vi "TakaData_TMotor_LightField.vi"(0 "Start position Y":dbl, 1 "Start position X":dbl, 2 "TotalSteps Y":i32, 3 "TotalSteps X":i32, 4 "Step Size Y":dbl, 5 "Step Size X":dbl, 7 "min":i32, 9 "max":i32, 10 "TCubeDCServoControl Y":refnum<k24>(container), 12 "TCubeDCServoControl X":refnum<k24>(container), 13 "TOTAL STOP":bool, 19 "Take data":bool) -> (14 "Intensity Graph":dbl[][](graph), 15 "ROI 1, Frame 1, Row 1":dbl[](graph), 16 "Data":T1(array[cluster]))   [LabVIEW 2020]
uses:
  D:/Programs/Fatima/Lightfield-LabVIEW Automation/lightfield-automation-labview/TCube_motion/Kinesis/Thorlabs.MotionControl.Controls.dll
  Kinesis/Thorlabs.MotionControl.Controls.dll
  D:/Programs/Fatima/Lightfield-LabVIEW Automation/lightfield-automation-labview/TCube_motion/Kinesis/Thorlabs.MotionControl.TCube.DCServoCLI.dll
  Kinesis/Thorlabs.MotionControl.TCube.DCServoCLI.dll
  <vilib>/express/express shared/transition.llb/Dynamic To Waveform Array.vi
  <vilib>/express/express signal manip/GetorSetDDTAttributes/Set DDT Attributes/SetT0.vi
  <vilib>/express/express shared/transition.llb/Waveform Array To Dynamic.vi
  <vilib>/express/express signal manip/GetorSetDDTAttributes/Set DDT Attributes/Set DDT Properties.xnode
  LightField Automation.lvclass
panel:
  out "Sums array":dbl[][](array[numeric])
  out "final":dbl[][](array[numeric])
  out "Position Y":i32
  out "Position X":i32
  out "Ys":dbl[](array[numeric])
  out "Xs":dbl[](array[numeric])
  out "sumas":dbl[](array[numeric])
  out "sum":dbl
  in  "SerialNumber X":string="83819717"
  in  "SerialNumber Y":string="83817852"
  # "Range"
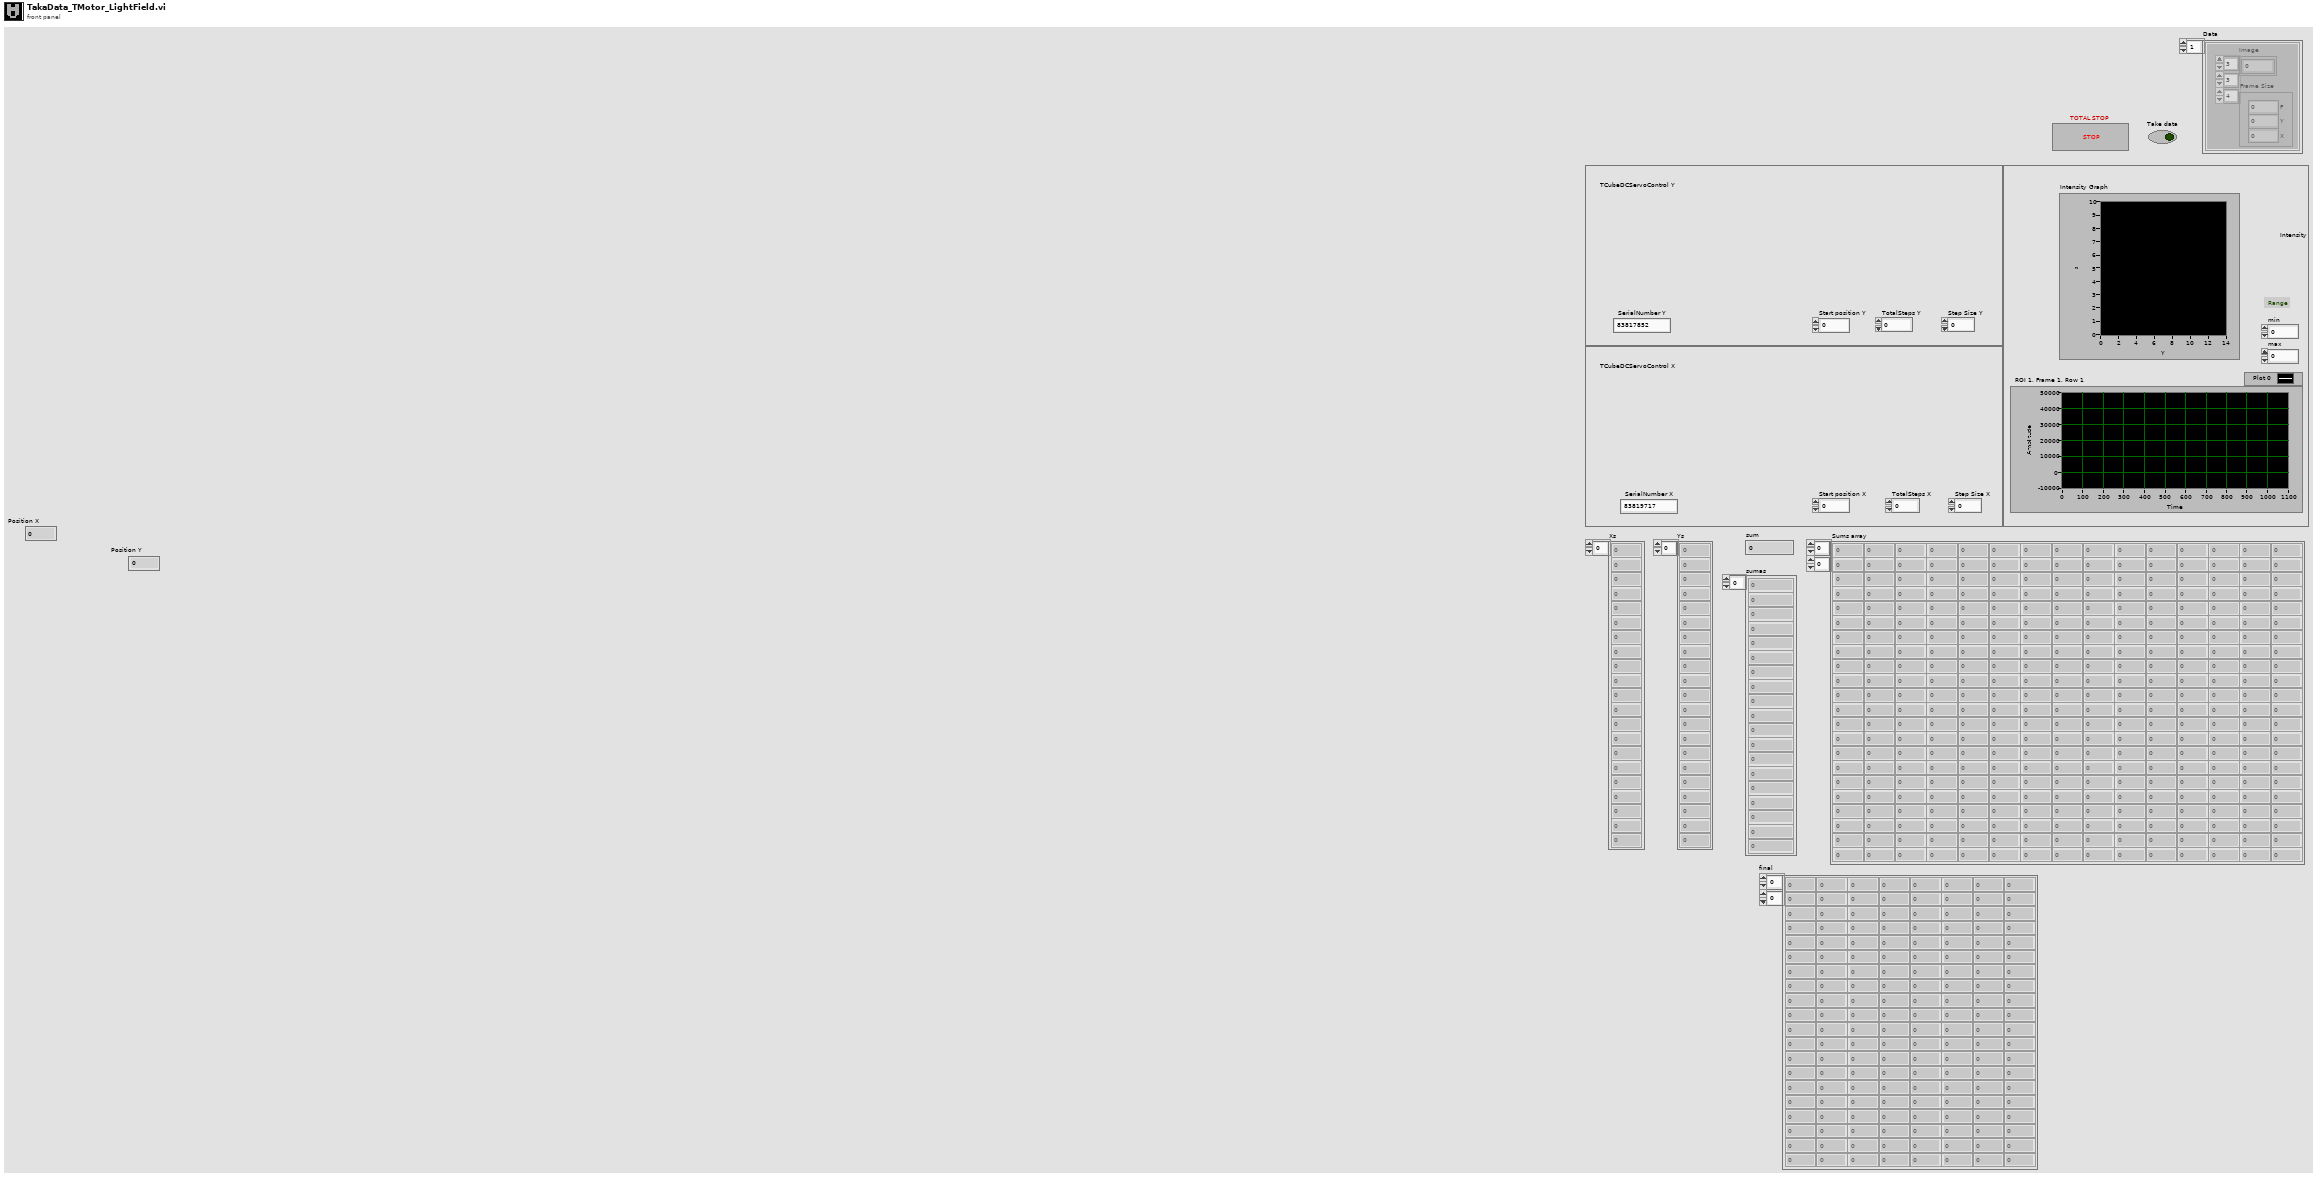
[diagram p1: front panel]
types:
  T1 = cluster{"Image":dbl[][][], "Frame Size":cluster{"F":i32, "Y":i32, "X":i32}}[]
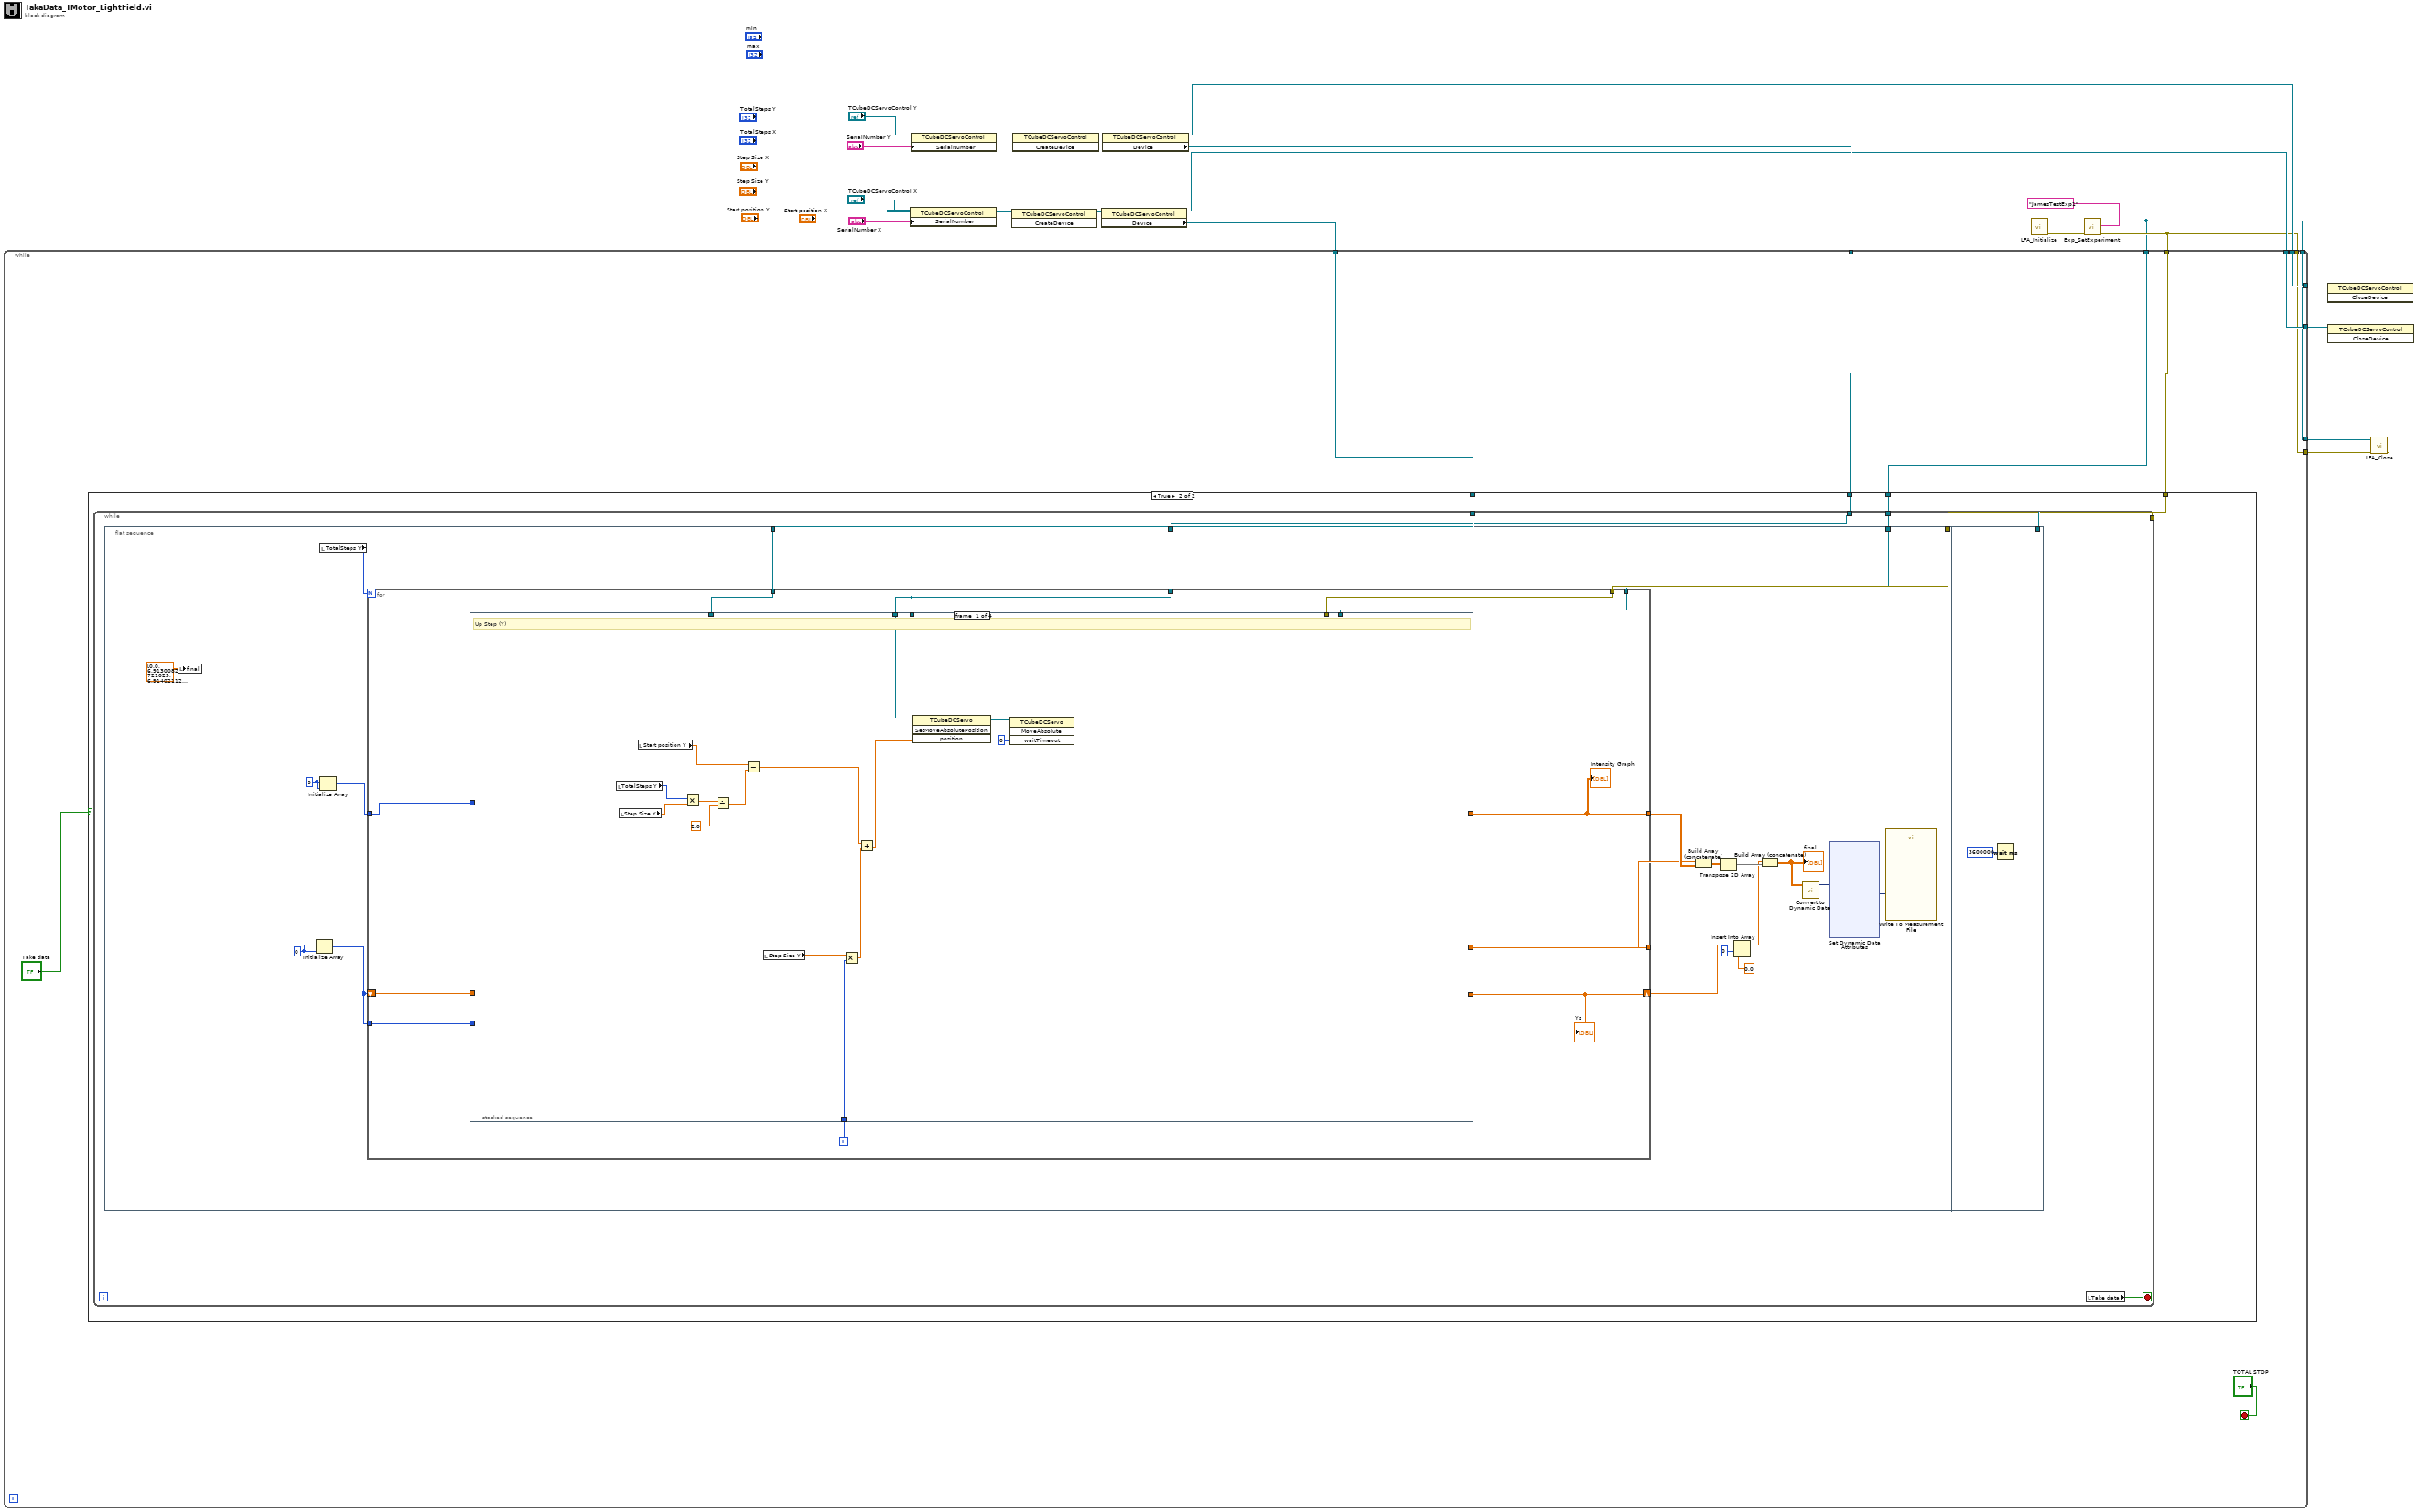
[diagram p0: block diagram]
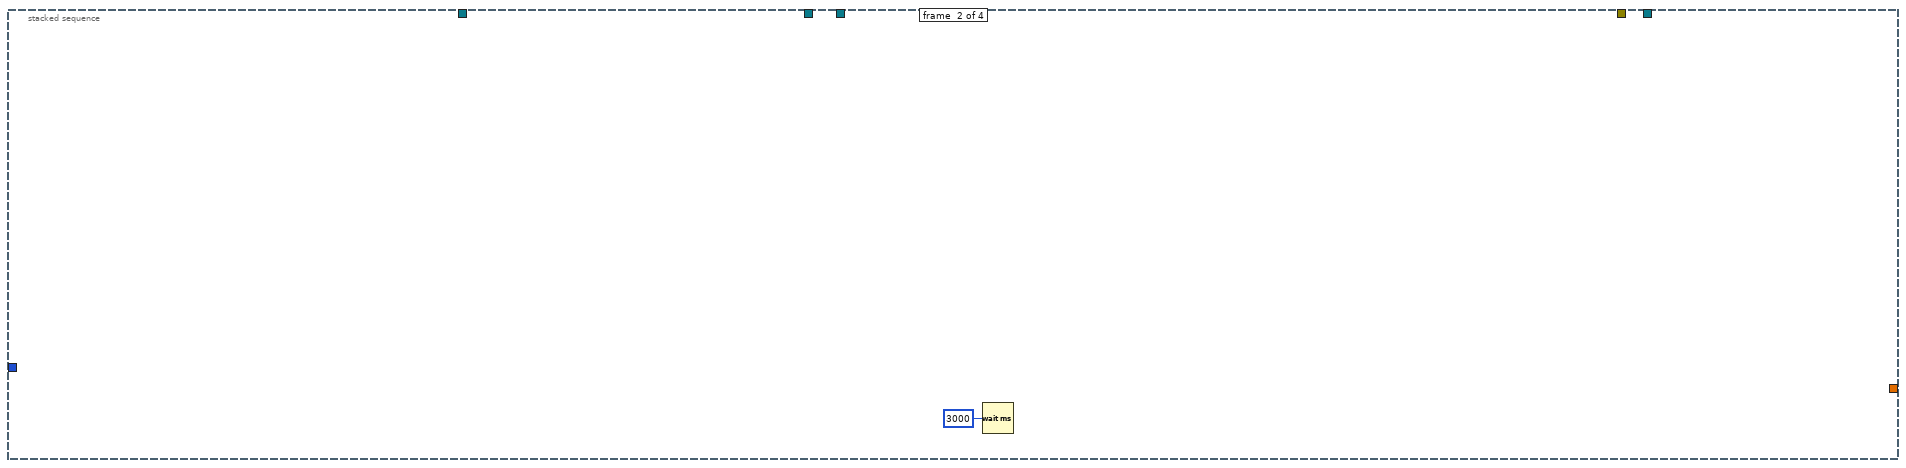
[diagram p3: hidden frame]
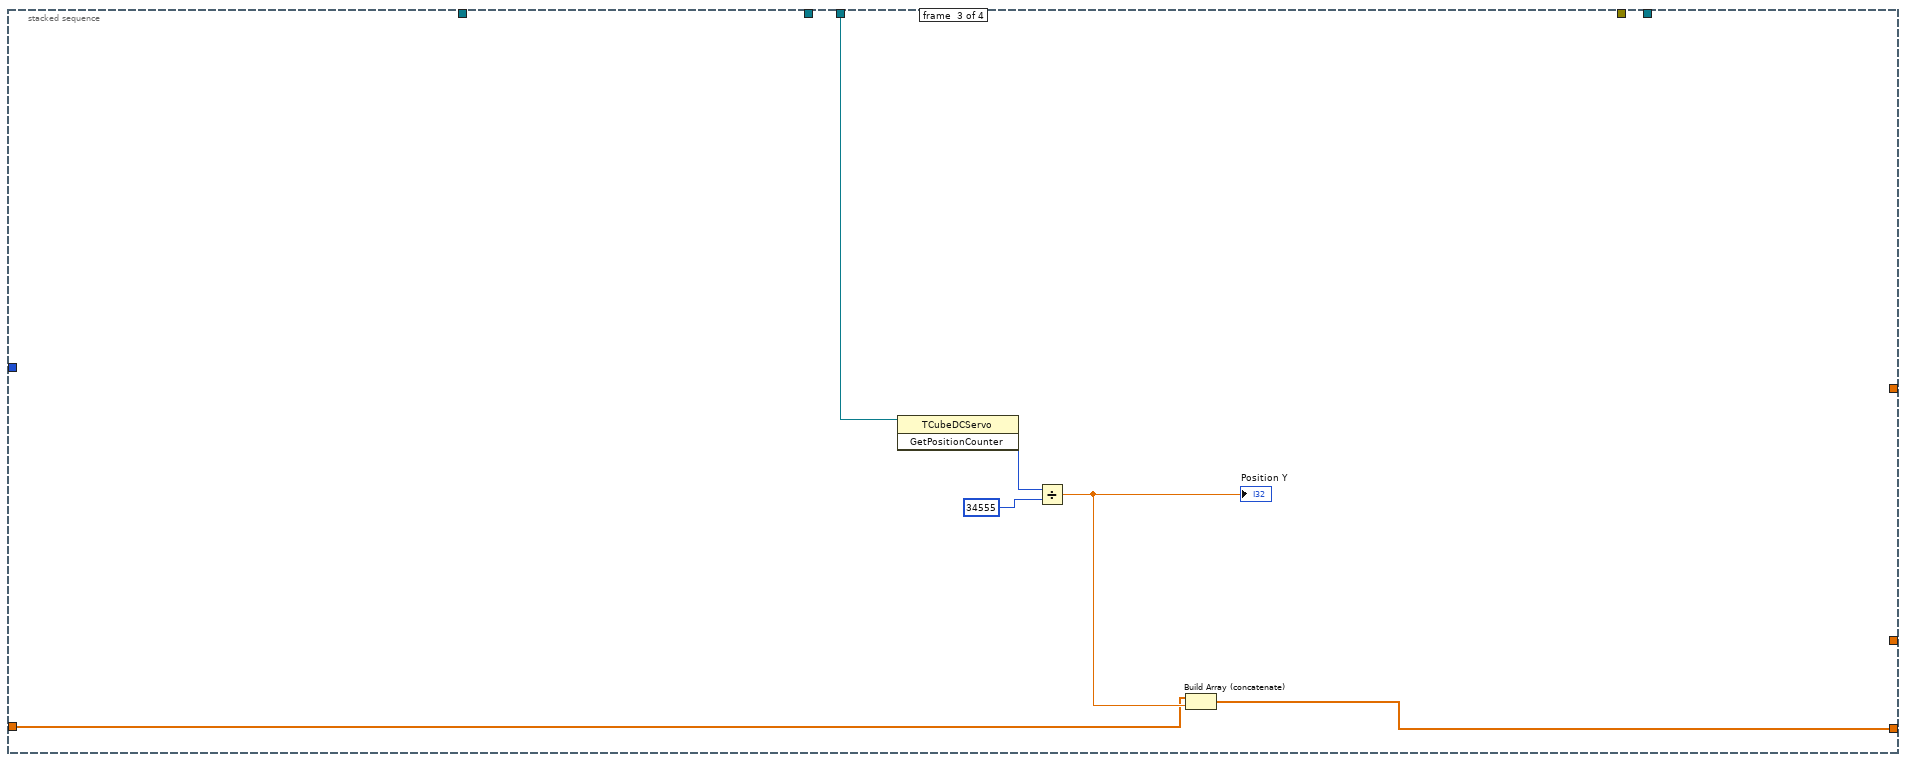
[diagram p4: hidden frame]
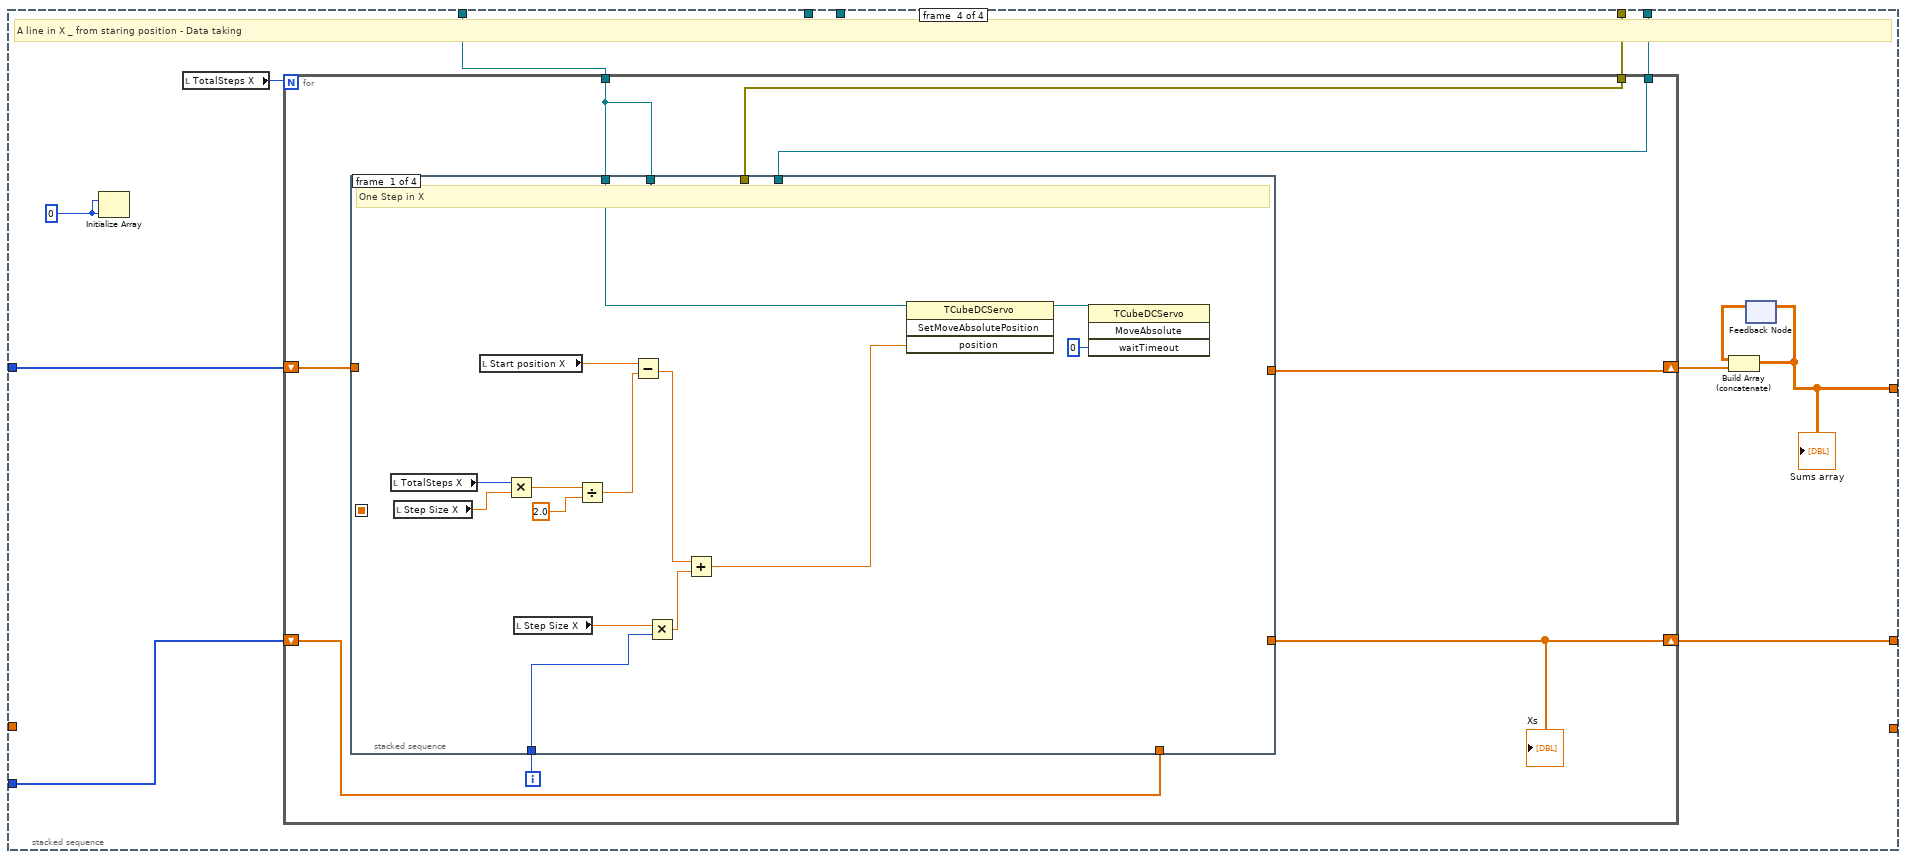
[diagram p5: hidden frame]
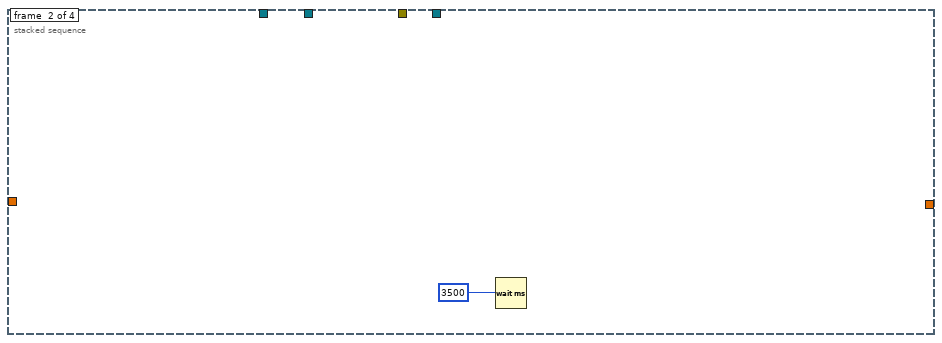
[diagram p6: hidden frame]
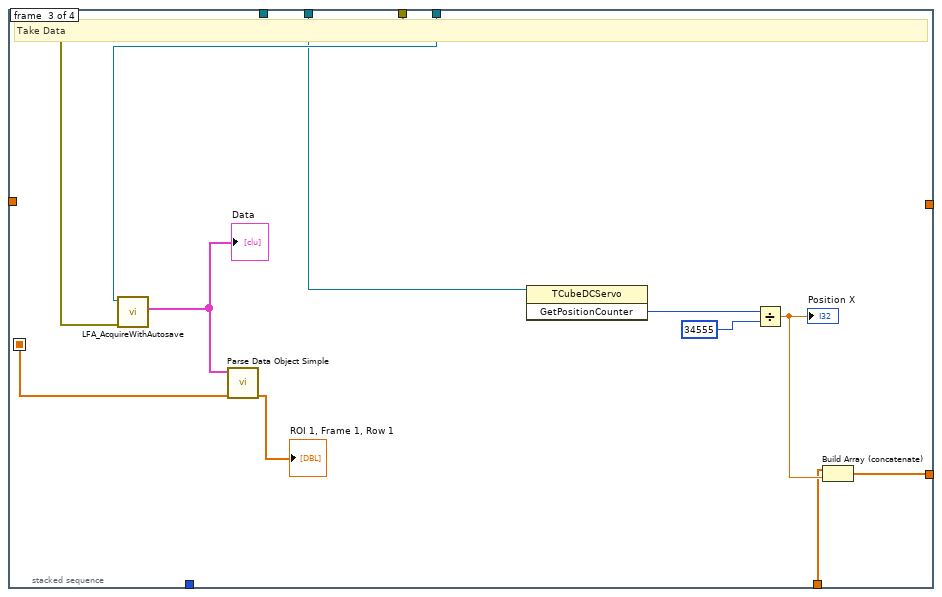
[diagram p7: hidden frame]
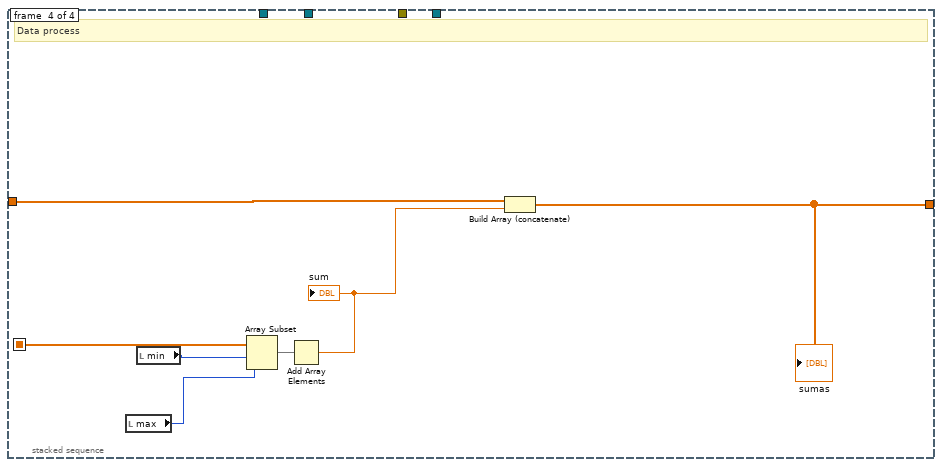
[diagram p8: hidden frame]
diagram:
  n1 = property class="TCubeDCServoControl"(reference="TCubeDCServoControl X", "SerialNumber"="SerialNumber X") -> (reference out=w16:refnum<k24>)  [unwired: 1 in, 1 out]
  n2 = property class="TCubeDCServoControl"(reference="TCubeDCServoControl Y", "SerialNumber"="SerialNumber Y") -> (reference out=w17:refnum<k24>)  [unwired: 1 in, 1 out]
  n3 = invoke class="TCubeDCServoControl" method="CreateDevice"(reference=w16) -> (reference out=w15:refnum<k24>)  [unwired: 2 in, 2 out]
  n4 = invoke class="TCubeDCServoControl" method="CreateDevice"(reference=w17) -> (reference out=w14:refnum<k24>)  [unwired: 2 in, 2 out]
  n5 = property class="TCubeDCServoControl"(reference=w15) -> (reference out=w11:refnum<k24>, "Device"=w13:refnum<k24>)  [unwired: 1 in, 1 out]
  n6 = property class="TCubeDCServoControl"(reference=w14) -> (reference out=w10:refnum<k24>, "Device"=w12:refnum<k24>)  [unwired: 1 in, 1 out]
  n7 = call "LFA_Initialize.vi"() -> ("error out"=w7:errorcluster, "LightField Automation out"=w6:refnum<class "LightField Automation.lvclass">)  [unwired: 10 in]
  n8 = call "Exp_SetExperiment.vi"("error in (no error)"=w7, "ExperimentName"="JamesTestExp1", "LightField Automation in"=w6) -> ("error out"=w4:errorcluster, "LightField Automation out"=w2:refnum<class "LightField Automation.lvclass">)  [unwired: 7 in]
  n9 = while {
    tunnel: w13 -> [w31]
    tunnel: w12 -> [w30]
    tunnel: w11 -> [w27]
    tunnel: w10 -> [w28]
    tunnel: [w28] -> w9
    tunnel: [w27] -> w8
    tunnel: w4 -> [w26]
    tunnel: w2 -> [w25]
    tunnel: [w24] -> w3
    tunnel: w4 -> [w24]
    tunnel: w2 -> [w23]
    tunnel: [w23] -> w1
    stop <- "TOTAL STOP" stop-if-true
    n10 = case shown="True" "Take data" {
      tunnel: w31 -> [_ w35]
      tunnel: w30 -> [_ w34]
      tunnel: w26 -> [_ w33]
      tunnel: w25 -> [_ w32]
      frame False {
      }
      frame True {
        n11 = while {
          tunnel: w35 -> [w40]
          tunnel: w34 -> [w39]
          tunnel: w33 -> [w38]
          tunnel: w32 -> [w37]
          stop <- w36 stop-if-true
          n12 = flat-sequence {
            tunnel: w40 -> [w61]
            tunnel: w39 -> [w60]
            tunnel: w38 -> [w43]
            tunnel: w37 -> [w42]
            tunnel: w39 -> [_]
            frame #0 {
              n13 = local write "final"(dbl[][] [[0.0, 6.913008247721025, 6.914021125741572, 6.905034003762118, 0.0, 0.0, 0.0, 0.0, 0.0, 0.0, 0.0, 0.0, 0.0, 0.0, 0.0, 0.0, 0.0, 0.0, 0.0, 0.0, 0.0, 0.0, 0.0, 0.0, 0.0, 0.0, 0.0, 0.0, 0.0, 0.0, 0.0, 0.0, 0.0, 0.0, 0.0, 0.0, 0.0, 0.0, 0.0, 0.0, 0.0, 0.0, 0.0, 0.0, 0.0, 0.0, 0.0, 0.0, 0.0], [1.5549992765156997, 544812.0, 544090.0, 545179.0, 545715.0, 514333.0, 540922.0, 542396.0, 542285.0, 540560.0, 539039.0, 510424.0, 540195.0, 540314.0, 541219.0, 540298.0, 539937.0, 540241.0, 544096.0, 540073.0, 545582.0, 546887.0, 547871.0, 543433.0, 548007.0, 542981.0, 957208.0, 926352.0, 905747.0, 922784.0, 904990.0, 870993.0, 910759.0, 903241.0, 906709.0, 908407.0, 903081.0, 894363.0, 895956.0, 885081.0, 878868.0, 868923.0, 860345.0, 860164.0, 414099.0, 832984.0, 915964.0, 915550.0, 913612.0], [1.5560121545362466, 545733.0, 544067.0, 545727.0, 546383.0, 540108.0, 542618.0, 541416.0, 541921.0, 541366.0, 549097.0, 540069.0, 541798.0, 541787.0, 541735.0, 541061.0, 540551.0, 540169.0, 543322.0, 540985.0, 546990.0, 547753.0, 546419.0, 541791.0, 548732.0, 543701.0, 993802.0, 946737.0, 971731.0, 951934.0, 915910.0, 906974.0, 907656.0, 905532.0, 906209.0, 903123.0, 897827.0, 892981.0, 888670.0, 874667.0, 871177.0, 857388.0, 850453.0, 852206.0, 844420.0, 830700.0, 948486.0, 950227.0, 949317.0], [1.556996093184778, 544155.0, 546607.0, 545261.0, 545747.0, 539580.0, 541161.0, 541772.0, 542512.0, 542112.0, 543649.0, 542433.0, 541919.0, 540621.0, 541770.0, 540502.0, 540316.0, 539855.0, 544925.0, 540392.0, 548195.0, 548882.0, 547832.0, 543029.0, 547228.0, 542787.0, 1000807.0, 978724.0, 947276.0, 922920.0, 900298.0, 895935.0, 902551.0, 904790.0, 909566.0, 903382.0, 893688.0, 882872.0, 883549.0, 876666.0, 864023.0, 414189.0, 845327.0, 839020.0, 843953.0, 827653.0, 982771.0, 983665.0, 977361.0], [1.5580089712053249, 544427.0, 544994.0, 545470.0, 546088.0, 539467.0, 541280.0, 541335.0, 541435.0, 542389.0, 547198.0, 541142.0, 541888.0, 540202.0, 540849.0, 541026.0, 539733.0, 539755.0, 544403.0, 535495.0, 547303.0, 547477.0, 547597.0, 503588.0, 546503.0, 543616.0, 966404.0, 925525.0, 904488.0, 893014.0, 885574.0, 897442.0, 904190.0, 906296.0, 909538.0, 905421.0, 893034.0, 880657.0, 877884.0, 864949.0, 860249.0, 854976.0, 840735.0, 819745.0, 826272.0, 812048.0, 996291.0, 972438.0, 935385.0], [1.5589929098538562, 545797.0, 545078.0, 546072.0, 546267.0, 537641.0, 540581.0, 542198.0, 542024.0, 540765.0, 543910.0, 541820.0, 540495.0, 541376.0, 541507.0, 540651.0, 541107.0, 540726.0, 544873.0, 539918.0, 547002.0, 548019.0, 548041.0, 546450.0, 547549.0, 541492.0, 916359.0, 897407.0, 889874.0, 893440.0, 891676.0, 905513.0, 894018.0, 908382.0, 910573.0, 906943.0, 895279.0, 883247.0, 874418.0, 863211.0, 856330.0, 854683.0, 840472.0, 814710.0, 816400.0, 806592.0, 956806.0, 921714.0, 906893.0], [1.5600057878744031, 544957.0, 543946.0, 544874.0, 546580.0, 538437.0, 542109.0, 541565.0, 541801.0, 541685.0, 539016.0, 541010.0, 541661.0, 541347.0, 541562.0, 541000.0, 540791.0, 540575.0, 543424.0, 533735.0, 546273.0, 548535.0, 549166.0, 547468.0, 546940.0, 542153.0, 900486.0, 892485.0, 893499.0, 896645.0, 893078.0, 897208.0, 911867.0, 906956.0, 910577.0, 905937.0, 892721.0, 859617.0, 873066.0, 865224.0, 854881.0, 850148.0, 846279.0, 826805.0, 824677.0, 815990.0, 906877.0, 898108.0, 899080.0], [1.5609897265229344, 544895.0, 545149.0, 545840.0, 546859.0, 538372.0, 542964.0, 541471.0, 541018.0, 541608.0, 540553.0, 541758.0, 541280.0, 541605.0, 542239.0, 541908.0, 540514.0, 540450.0, 545392.0, 536001.0, 547854.0, 548794.0, 548208.0, 546566.0, 547851.0, 549415.0, 901658.0, 887451.0, 898081.0, 895266.0, 893039.0, 901155.0, 907181.0, 905206.0, 908855.0, 902076.0, 896759.0, 901383.0, 875270.0, 861471.0, 852212.0, 849333.0, 857402.0, 847508.0, 855392.0, 850490.0, 899566.0, 901543.0, 902029.0], [1.5620026045434814, 545176.0, 544361.0, 545016.0, 545059.0, 539403.0, 541973.0, 541930.0, 540981.0, 541461.0, 539898.0, 540606.0, 540336.0, 539776.0, 541040.0, 541423.0, 540713.0, 540599.0, 545524.0, 529378.0, 545787.0, 548520.0, 530786.0, 547217.0, 548115.0, 547737.0, 903147.0, 891251.0, 898795.0, 898663.0, 892796.0, 907311.0, 910510.0, 906770.0, 907801.0, 898624.0, 895068.0, 897240.0, 874273.0, 868222.0, 860063.0, 852777.0, 867950.0, 876942.0, 874606.0, 868711.0, 897961.0, 903725.0, 905170.0], [1.5629865431920127, 336173.0, 545567.0, 546431.0, 546821.0, 530129.0, 542537.0, 541161.0, 540768.0, 542160.0, 541439.0, 540999.0, 542117.0, 541843.0, 542614.0, 540392.0, 540853.0, 540313.0, 543673.0, 499165.0, 545984.0, 548073.0, 537798.0, 548591.0, 546998.0, 548780.0, 907838.0, 891732.0, 901308.0, 898026.0, 892739.0, 903169.0, 911446.0, 907353.0, 907261.0, 896720.0, 892783.0, 896372.0, 877559.0, 866276.0, 864710.0, 855235.0, 873679.0, 889080.0, 870095.0, 834179.0, 902021.0, 907248.0, 905191.0], [1.5639994212125596, 545415.0, 545849.0, 544890.0, 545734.0, 542044.0, 541843.0, 541342.0, 542062.0, 541454.0, 541551.0, 541101.0, 541085.0, 542151.0, 541013.0, 539085.0, 539718.0, 531837.0, 540436.0, 543617.0, 546609.0, 547981.0, 542058.0, 548618.0, 496892.0, 547803.0, 912725.0, 850046.0, 905669.0, 902124.0, 896849.0, 898399.0, 914550.0, 909252.0, 906642.0, 893078.0, 883576.0, 887001.0, 871714.0, 858905.0, 864502.0, 856973.0, 877401.0, 898022.0, 879924.0, 895045.0, 906393.0, 911175.0, 907999.0], [1.5650122992331066, 0.0, 0.0, 0.0, 0.0, 0.0, 0.0, 0.0, 0.0, 0.0, 0.0, 0.0, 0.0, 0.0, 0.0, 0.0, 0.0, 0.0, 0.0, 0.0, 0.0, 0.0, 0.0, 0.0, 0.0, 0.0, 912697.0, 853203.0, 905078.0, 901656.0, 899447.0, 905117.0, 918626.0, 912774.0, 905335.0, 891192.0, 880762.0, 883225.0, 872482.0, 862083.0, 855974.0, 854460.0, 870701.0, 889213.0, 874501.0, 894669.0, 909913.0, 912967.0, 911442.0], [1.5659962378816379, 0.0, 0.0, 0.0, 0.0, 0.0, 0.0, 0.0, 0.0, 0.0, 0.0, 0.0, 0.0, 0.0, 0.0, 0.0, 0.0, 0.0, 0.0, 0.0, 0.0, 0.0, 0.0, 0.0, 0.0, 0.0, 900230.0, 794504.0, 899512.0, 897560.0, 899060.0, 903923.0, 898265.0, 913246.0, 898893.0, 877900.0, 871302.0, 875382.0, 875734.0, 870605.0, 852610.0, 852644.0, 863529.0, 874320.0, 874581.0, 884633.0, 908558.0, 909935.0, 911095.0], [1.5670091159021848, 0.0, 0.0, 0.0, 0.0, 0.0, 0.0, 0.0, 0.0, 0.0, 0.0, 0.0, 0.0, 0.0, 0.0, 0.0, 0.0, 0.0, 0.0, 0.0, 0.0, 0.0, 0.0, 0.0, 0.0, 0.0, 898150.0, 883779.0, 891737.0, 891311.0, 892229.0, 871876.0, 904014.0, 906225.0, 879453.0, 863541.0, 861575.0, 866968.0, 875231.0, 876673.0, 867543.0, 857713.0, 860505.0, 858533.0, 858223.0, 867816.0, 903650.0, 899995.0, 901363.0], [1.5679930545507164, 0.0, 0.0, 0.0, 0.0, 0.0, 0.0, 0.0, 0.0, 0.0, 0.0, 0.0, 0.0, 0.0, 0.0, 0.0, 0.0, 0.0, 0.0, 0.0, 0.0, 0.0, 0.0, 0.0, 0.0, 0.0, 899923.0, 877984.0, 892189.0, 890054.0, 885407.0, 893213.0, 895135.0, 898762.0, 872617.0, 852275.0, 846627.0, 855610.0, 860540.0, 870540.0, 874446.0, 867953.0, 864715.0, 849073.0, 838829.0, 857485.0, 900004.0, 900763.0, 898308.0], [1.5690059325712633, 0.0, 0.0, 0.0, 0.0, 0.0, 0.0, 0.0, 0.0, 0.0, 0.0, 0.0, 0.0, 0.0, 0.0, 0.0, 0.0, 0.0, 0.0, 0.0, 0.0, 0.0, 0.0, 0.0, 0.0, 0.0, 900049.0, 878818.0, 893092.0, 850492.0, 883727.0, 872055.0, 886336.0, 883052.0, 865029.0, 848803.0, 850586.0, 852654.0, 851858.0, 864331.0, 872776.0, 870413.0, 880211.0, 854698.0, 812935.0, 852028.0, 911383.0, 899029.0, 898690.0], [1.5699898712197946, 0.0, 0.0, 0.0, 0.0, 0.0, 0.0, 0.0, 0.0, 0.0, 0.0, 0.0, 0.0, 0.0, 0.0, 0.0, 0.0, 0.0, 0.0, 0.0, 0.0, 0.0, 0.0, 0.0, 0.0, 0.0, 902955.0, 879976.0, 899283.0, 895768.0, 884736.0, 866045.0, 866242.0, 869188.0, 855707.0, 855217.0, 856095.0, 857336.0, 857833.0, 858578.0, 862626.0, 869801.0, 858111.0, 871991.0, 848077.0, 856437.0, 904011.0, 899786.0, 900983.0], [1.5710027492403416, 0.0, 0.0, 0.0, 0.0, 0.0, 0.0, 0.0, 0.0, 0.0, 0.0, 0.0, 0.0, 0.0, 0.0, 0.0, 0.0, 0.0, 0.0, 0.0, 0.0, 0.0, 0.0, 0.0, 0.0, 0.0, 899155.0, 881833.0, 897840.0, 901034.0, 891551.0, 867202.0, 855374.0, 860312.0, 858351.0, 862323.0, 860043.0, 860337.0, 860736.0, 859479.0, 861496.0, 869480.0, 894063.0, 888501.0, 870096.0, 868012.0, 904494.0, 905187.0, 905371.0], [1.5719866878888729, 0.0, 0.0, 0.0, 0.0, 0.0, 0.0, 0.0, 0.0, 0.0, 0.0, 0.0, 0.0, 0.0, 0.0, 0.0, 0.0, 0.0, 0.0, 0.0, 0.0, 0.0, 0.0, 0.0, 0.0, 0.0, 887679.0, 872395.0, 892984.0, 898344.0, 892930.0, 878847.0, 851729.0, 861118.0, 866658.0, 868591.0, 858145.0, 855744.0, 852097.0, 860173.0, 871331.0, 880479.0, 895467.0, 894341.0, 886979.0, 888001.0, 899105.0, 903306.0, 903996.0], [1.5729995659094198, 0.0, 0.0, 0.0, 0.0, 0.0, 0.0, 0.0, 0.0, 0.0, 0.0, 0.0, 0.0, 0.0, 0.0, 0.0, 0.0, 0.0, 0.0, 0.0, 0.0, 0.0, 0.0, 0.0, 0.0, 0.0, 853315.0, 847512.0, 888874.0, 893244.0, 892566.0, 885785.0, 801973.0, 860507.0, 866622.0, 870234.0, 853549.0, 853090.0, 854914.0, 854906.0, 875579.0, 893984.0, 846541.0, 889392.0, 882226.0, 892030.0, 876413.0, 890775.0, 897971.0], [1.5740124439299668, 0.0, 0.0, 0.0, 0.0, 0.0, 0.0, 0.0, 0.0, 0.0, 0.0, 0.0, 0.0, 0.0, 0.0, 0.0, 0.0, 0.0, 0.0, 0.0, 0.0, 0.0, 0.0, 0.0, 0.0, 0.0, 838459.0, 826063.0, 875751.0, 883533.0, 882362.0, 876724.0, 850383.0, 856585.0, 868739.0, 877559.0, 866754.0, 861394.0, 856368.0, 850345.0, 877837.0, 900407.0, 900707.0, 883502.0, 867827.0, 890667.0, 845982.0, 869911.0, 893765.0], [1.574996382578498, 0.0, 0.0, 0.0, 0.0, 0.0, 0.0, 0.0, 0.0, 0.0, 0.0, 0.0, 0.0, 0.0, 0.0, 0.0, 0.0, 0.0, 0.0, 0.0, 0.0, 0.0, 0.0, 0.0, 0.0, 0.0, 812489.0, 809503.0, 861080.0, 874961.0, 876059.0, 860865.0, 859584.0, 862178.0, 866724.0, 879212.0, 873189.0, 865713.0, 859463.0, 855320.0, 873664.0, 896550.0, 895263.0, 873242.0, 859861.0, 883140.0, 840536.0, 854125.0, 880926.0], [1.576009260599045, 0.0, 0.0, 0.0, 0.0, 0.0, 0.0, 0.0, 0.0, 0.0, 0.0, 0.0, 0.0, 0.0, 0.0, 0.0, 0.0, 0.0, 0.0, 0.0, 0.0, 0.0, 0.0, 0.0, 0.0, 0.0, 851818.0, 794983.0, 839516.0, 858340.0, 862512.0, 858296.0, 875210.0, 865789.0, 860037.0, 870684.0, 872801.0, 879759.0, 864398.0, 867539.0, 874982.0, 888241.0, 877631.0, 863713.0, 845486.0, 885909.0, 846425.0, 834439.0, 859576.0], [1.5769931992475763, 0.0, 0.0, 0.0, 0.0, 0.0, 0.0, 0.0, 0.0, 0.0, 0.0, 0.0, 0.0, 0.0, 0.0, 0.0, 0.0, 0.0, 0.0, 0.0, 0.0, 0.0, 0.0, 0.0, 0.0, 0.0, 845660.0, 799921.0, 824126.0, 820343.0, 845675.0, 857053.0, 874803.0, 873615.0, 861408.0, 860003.0, 862092.0, 878552.0, 870005.0, 874566.0, 884010.0, 873435.0, 859821.0, 849576.0, 839723.0, 887722.0, 850691.0, 824924.0, 838242.0], [1.5780060772681233, 0.0, 0.0, 0.0, 0.0, 0.0, 0.0, 0.0, 0.0, 0.0, 0.0, 0.0, 0.0, 0.0, 0.0, 0.0, 0.0, 0.0, 0.0, 0.0, 0.0, 0.0, 0.0, 0.0, 0.0, 0.0, 838458.0, 803968.0, 820039.0, 802330.0, 823535.0, 836657.0, 879299.0, 879696.0, 862522.0, 846809.0, 838297.0, 862995.0, 856255.0, 872603.0, 889252.0, 865758.0, 849942.0, 846346.0, 839732.0, 880025.0, 848443.0, 829737.0, 825550.0], [1.5789900159166546, 0.0, 0.0, 0.0, 0.0, 0.0, 0.0, 0.0, 0.0, 0.0, 0.0, 0.0, 0.0, 0.0, 0.0, 0.0, 0.0, 0.0, 0.0, 0.0, 0.0, 0.0, 0.0, 0.0, 0.0, 0.0, 824182.0, 799501.0, 821379.0, 801283.0, 825077.0, 838329.0, 863788.0, 870684.0, 855236.0, 837890.0, 816819.0, 839553.0, 847048.0, 864015.0, 894582.0, 872354.0, 833986.0, 839739.0, 860968.0, 877590.0, 840730.0, 830841.0, 826878.0], [1.5800028939372015, 0.0, 0.0, 0.0, 0.0, 0.0, 0.0, 0.0, 0.0, 0.0, 0.0, 0.0, 0.0, 0.0, 0.0, 0.0, 0.0, 0.0, 0.0, 0.0, 0.0, 0.0, 0.0, 0.0, 0.0, 0.0, 824964.0, 795837.0, 815097.0, 808024.0, 831421.0, 846746.0, 846660.0, 852057.0, 837469.0, 834622.0, 819140.0, 830413.0, 839410.0, 846662.0, 883230.0, 867443.0, 833234.0, 836675.0, 845173.0, 860473.0, 830543.0, 828873.0, 823869.0], [1.5809868325857328, 0.0, 0.0, 0.0, 0.0, 0.0, 0.0, 0.0, 0.0, 0.0, 0.0, 0.0, 0.0, 0.0, 0.0, 0.0, 0.0, 0.0, 0.0, 0.0, 0.0, 0.0, 0.0, 0.0, 0.0, 0.0, 830361.0, 788771.0, 808671.0, 802703.0, 838543.0, 850689.0, 845538.0, 828206.0, 824275.0, 829734.0, 822489.0, 849025.0, 837964.0, 832115.0, 856696.0, 851028.0, 826729.0, 832160.0, 818624.0, 852220.0, 824672.0, 825485.0, 818602.0], [1.5819997106062798, 0.0, 0.0, 0.0, 0.0, 0.0, 0.0, 0.0, 0.0, 0.0, 0.0, 0.0, 0.0, 0.0, 0.0, 0.0, 0.0, 0.0, 0.0, 0.0, 0.0, 0.0, 0.0, 0.0, 0.0, 0.0, 833107.0, 794138.0, 805009.0, 776996.0, 815824.0, 854813.0, 848376.0, 823622.0, 813702.0, 825955.0, 821209.0, 845858.0, 833977.0, 820258.0, 827807.0, 835229.0, 825721.0, 828832.0, 823507.0, 847929.0, 829986.0, 819382.0, 812699.0], [1.5830125886268267, 0.0, 0.0, 0.0, 0.0, 0.0, 0.0, 0.0, 0.0, 0.0, 0.0, 0.0, 0.0, 0.0, 0.0, 0.0, 0.0, 0.0, 0.0, 0.0, 0.0, 0.0, 0.0, 0.0, 0.0, 0.0, 834138.0, 800682.0, 808091.0, 770002.0, 793107.0, 844032.0, 846347.0, 825928.0, 811744.0, 820808.0, 828026.0, 830245.0, 827102.0, 812182.0, 813935.0, 823819.0, 827937.0, 835794.0, 821444.0, 838266.0, 835231.0, 821151.0, 811092.0], [1.5839965272753582, 0.0, 0.0, 0.0, 0.0, 0.0, 0.0, 0.0, 0.0, 0.0, 0.0, 0.0, 0.0, 0.0, 0.0, 0.0, 0.0, 0.0, 0.0, 0.0, 0.0, 0.0, 0.0, 0.0, 0.0, 0.0, 807007.0, 804348.0, 817194.0, 773514.0, 787109.0, 802104.0, 835007.0, 820473.0, 811838.0, 824253.0, 838614.0, 829894.0, 810918.0, 801837.0, 806735.0, 818216.0, 831857.0, 834292.0, 811343.0, 822804.0, 832845.0, 826133.0, 820344.0]] ("final")) -> ()
            }
            frame #1 {
              w56 = 0 ("dimension size")
              w58 = 0 ("dimension size")
              n14 = Initialize Array(w58, w58) -> (w57:i32[])
              n15 = local read "TotalSteps Y"() -> (w59:i32)
              n16 = Initialize Array "Initialize Array"(w56, w56) -> (w53:i32[])
              n17 = for {
                N: w59 -> [_]
                tunnel: w61 -> [w86]
                tunnel: w60 -> [w77]
                tunnel: w43 -> [w84]
                tunnel: w42 -> [w83]
                shift-right: [w81] -> w52
                shift-left: w57 -> [w82]
                tunnel: w57 -> [w80]
                tunnel: [w79] -> w47
                tunnel: w53 -> [w78]
                tunnel: [w76] -> w50
                i -> [w85]
                n18 = stacked-sequence {
                  tunnel: w85 -> [w97 _ _ _]
                  tunnel: w77 -> [w98 _ _ _]
                  tunnel: w86 -> [_ _ _ w118]
                  tunnel: w84 -> [_ _ _ w116]
                  tunnel: w83 -> [_ _ _ w115]
                  tunnel: w82 -> [_ _ w103 _]
                  tunnel: [_ _ w104 _] -> w81
                  tunnel: w80 -> [_ _ _ w114]
                  tunnel: [_ _ _ w112] -> w79
                  tunnel: w78 -> [_ _ _ w113]
                  tunnel: [_ _ _ w108] -> w76
                  tunnel: w77 -> [_ _ w102 _]
                  frame #0 {
                    # "Up Step (Y)"
                    n19 = local read "TotalSteps Y"() -> (w93:i32)
                    n20 = local read "Step Size Y"() -> (w92:dbl)
                    n21 = local read "Start position Y"() -> (w88:dbl)
                    n22 = Multiply(x=w93, y=w92) -> (x*y=w91:dbl)
                    n23 = Divide(x=w91, y=2.0) -> (x/y=w89:dbl)
                    n24 = Subtract(x=w88, y=w89) -> (x-y=w87:dbl)
                    n25 = local read "Step Size Y"() -> (w95:dbl)
                    n26 = Multiply(x=w95, y=w97) -> (x*y=w96:dbl)
                    n27 = Add(x=w87, y=w96) -> (x+y=w94:dbl)
                    n28 = invoke class="TCubeDCServo" method="SetMoveAbsolutePosition"(reference=w98, "position"=w94) -> (reference out=w100:refnum<k24>)  [unwired: 2 in, 3 out]
                    n29 = invoke class="TCubeDCServo" method="MoveAbsolute"(reference=w100, "waitTimeout"=0) -> ()  [unwired: 2 in, 4 out]
                  }
                  frame #1 {
                    n30 = Wait (ms)(milliseconds to wait=u32 3000) -> ()  [unwired: 1 out]
                  }
                  frame #2 {
                    n31 = invoke class="TCubeDCServo" method="GetPositionCounter"(reference=w102) -> ("GetPositionCounter"=w107:i32)  [unwired: 2 in, 2 out]
                    n32 = Divide(x=w107, y=34555) -> (x/y=w105:dbl)
                    "Position Y" <- w105
                    n33 = Build Array (concatenate)(w103, w105) -> (w104:dbl[])
                  }
                  frame #3 {
                    w111 = 0 ("dimension size")
                    # "A line in X _ from staring position - Data taking"
                    n34 = Initialize Array(w111, w111) -> ()  [unwired: 1 out]
                    n35 = local read "TotalSteps X"() -> (w117:i32)
                    n36 = for {
                      N: w117 -> [_]
                      tunnel: w118 -> [w119]
                      tunnel: w116 -> [w126]
                      tunnel: w115 -> [w125]
                      shift-right: [w120] -> w110
                      shift-left: w113 -> [w123]
                      shift-right: [w121] -> w112
                      shift-left: w114 -> [w122]
                      i -> [w124]
                      n37 = stacked-sequence {
                        seq-local: [_ _ w148 _] -> [_ _ _ w157]
                        tunnel: w119 -> [w140 _ _ _]
                        tunnel: w124 -> [w137 _ _ _]
                        tunnel: w126 -> [_ _ w151 _]
                        tunnel: w125 -> [_ _ w150 _]
                        tunnel: w123 -> [_ _ _ w155]
                        tunnel: [_ _ _ w154] -> w120
                        tunnel: w122 -> [_ _ w143 _]
                        tunnel: [_ _ w144 _] -> w121
                        tunnel: w119 -> [_ _ w142 _]
                        frame #0 {
                          # "One Step in X"
                          n38 = local read "TotalSteps X"() -> (w133:i32)
                          n39 = local read "Step Size X"() -> (w132:dbl)
                          n40 = local read "Start position X"() -> (w134:dbl)
                          n41 = Multiply(x=w133, y=w132) -> (x*y=w128:dbl)
                          n42 = local read "Step Size X"() -> (w136:dbl)
                          n43 = Divide(x=w128, y=2.0) -> (x/y=w127:dbl)
                          n44 = Subtract(x=w134, y=w127) -> (x-y=w131:dbl)
                          n45 = Multiply(x=w136, y=w137) -> (x*y=w135:dbl)
                          n46 = Add(x=w131, y=w135) -> (x+y=w130:dbl)
                          n47 = invoke class="TCubeDCServo" method="SetMoveAbsolutePosition"(reference=w140, "position"=w130) -> (reference out=w139:refnum<k24>)  [unwired: 2 in, 3 out]
                          n48 = invoke class="TCubeDCServo" method="MoveAbsolute"(reference=w139, "waitTimeout"=0) -> ()  [unwired: 2 in, 4 out]
                        }
                        frame #1 {
                          n49 = Wait (ms)(milliseconds to wait=u32 3500 ("millisecond timer value")) -> ()  [unwired: 1 out]
                        }
                        frame #2 {
                          # "Take Data"
                          n50 = call "LFA_AcquireWithAutosave.vi"("error in (no error)"=w151, "LightField Automation in"=w150) -> ("Data"=w149:T1)  [unwired: 7 in, 2 out]
                          "Data" <- w149
                          n51 = call "Parse Data Object Simple.vi"("Data"=w149) -> ("ROI 1, Frame 1, Row 1"=w148:dbl[])  [unwired: 9 in, 1 out]
                          "ROI 1, Frame 1, Row 1" <- w148
                          n52 = invoke class="TCubeDCServo" method="GetPositionCounter"(reference=w142) -> ("GetPositionCounter"=w147:i32)  [unwired: 2 in, 2 out]
                          n53 = Divide(x=w147, y=34555) -> (x/y=w145:dbl)
                          "Position X" <- w145
                          n54 = Build Array (concatenate)(w143, w145) -> (w144:dbl[])
                        }
                        frame #3 {
                          # "Data process"
                          n55 = local read "max"() -> (w152:i32)
                          n56 = local read "min"() -> (w153:i32)
                          n57 = Array Subset(array=w157, index=w153, length=w152) -> (w158:dbl[])
                          n58 = Add Array Elements(numeric array=w158) -> (sum=w156:dbl)
                          "sum" <- w156
                          n59 = Build Array (concatenate)(w155, w156) -> (w154:dbl[])
                          "sumas" <- w154
                        }
                      }
                      "Xs" <- w121
                    }
                    n60 = feedback #1() -> (w109:dbl[][])  [unwired: 1 in]
                    n61 = Build Array (concatenate)(w109, w110) -> (w108:dbl[][])
                    "Sums array" <- w108
                    n62 = feedback-in #1(w108) -> ()
                  }
                }
                "Ys" <- w81
                "Intensity Graph" <- w76
              }
              n63 = Build Array (concatenate)(w47, w50) -> (w51:dbl[][])
              n64 = Transpose 2D Array(2D array=w51) -> (transposed array=w49:dbl[][])
              n65 = Insert Into Array(array=w52, index=0, new element=0.0 ("new element/subarray")) -> (w48:dbl[])
              n66 = Build Array (concatenate)(w48, w49) -> (w44:dbl[][])
              "final" <- w44
              n67 = call "Convert to Dynamic Data"("2D Array"=w44) -> ("Dynamic Data Type"=w46:dynamicdata)  [unwired: 3 in]
              n68 = xnode "Set Dynamic Data Attributes"("Signals In"=w46) -> ("Signals Out"=w45:dynamicdata)  [unwired: 3 in, 1 out]
              n69 = call "Write To Measurement File"("Signals"=w45) -> ()  [unwired: 16 in, 3 out]
            }
            frame #2 {
              n70 = Wait (ms)(milliseconds to wait=u32 3600000) -> ()  [unwired: 1 out]
            }
          }
          n71 = local read "Take data"() -> (w36:bool)
        }
      }
    }
  }
  n72 = invoke class="TCubeDCServoControl" method="CloseDevice"(reference=w9) -> ()  [unwired: 2 in, 3 out]
  n73 = invoke class="TCubeDCServoControl" method="CloseDevice"(reference=w8) -> ()  [unwired: 2 in, 3 out]
  n74 = call "LFA_Close.vi"("error in (no error)"=w3, "LightField Automation in"=w1) -> ()  [unwired: 8 in, 2 out]
